vi "Debug Flags.vi"(4 "Error In":errorcluster, 6 "Function":enum16{"Read", "Write"}(ring), 7 "Trace Flags In":bool[](array[boolean])) -> (0 "Error Out":errorcluster, 3 "Trace Flags Out":bool[](array[boolean]))   [LabVIEW 2014, in "Debugging.lvlib"]
uses:
  Debugging.lvlib
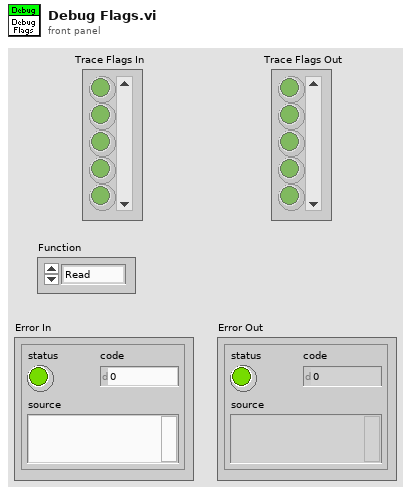
[diagram p1: front panel]
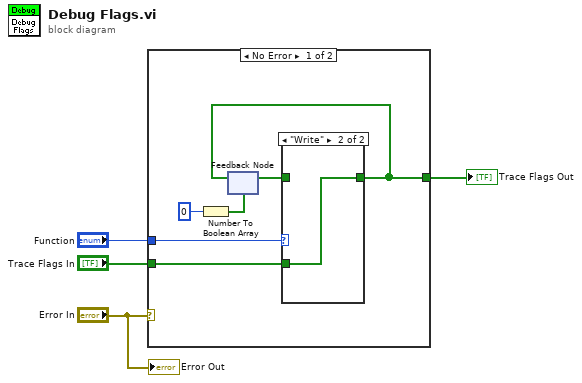
[diagram p0: block diagram]
diagram:
  n1 = case shown="No Error" "Error In" {
    tunnel: [w9 _] -> w4
    tunnel: "Function" -> [w8 _]
    tunnel: "Trace Flags In" -> [w7 _]
    frame No Error {
      n2 = Number To Boolean Array(number=u32 0) -> (Boolean array=w5:bool[])
      n3 = feedback #1(w5) -> (w10:bool[])
      n4 = case shown="\"Write\"" w8 {
        tunnel: [w11 w12] -> w9
        tunnel: w10 -> [w11 _]
        tunnel: w7 -> [_ w12]
        frame "Read" {
        }
        frame "Write" {
        }
      }
      n5 = feedback-in #1(w9) -> ()
    }
    frame Error {
    }
  }
  "Trace Flags Out" <- w4
  "Error Out" <- "Error In"
